vi "Check Main Measurement for Instrument Drivers.vi"(0 "Instrument containing subVIs":path[](array[path]), 5 "Measurement path":path, 11 "error in (no error)":errorcluster) -> (4 "Instrument containing subVIs Out":path[](array[path]), 15 "error out":errorcluster)   [LabVIEW 2021, in "Multiple Converter.lvlib"]
uses:
  Multiple Converter.lvlib
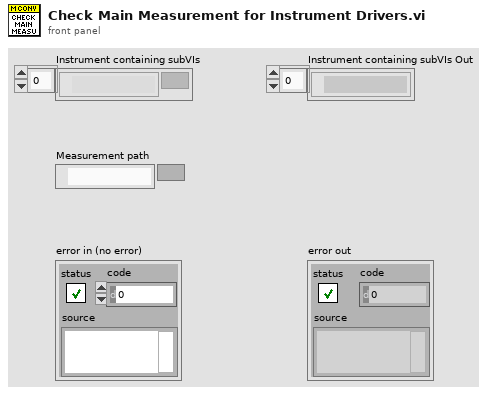
[diagram p1: front panel]
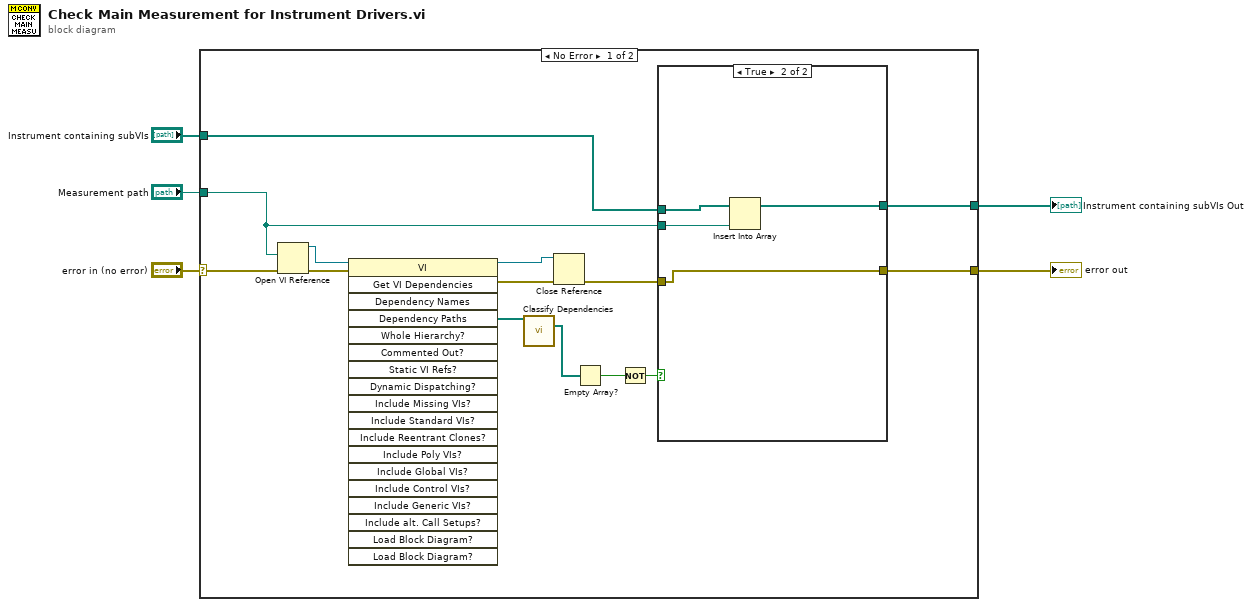
[diagram p0: block diagram]
diagram:
  n1 = case shown="No Error" "error in (no error)" {
    selector: "error in (no error)" -> [w16 w26]
    tunnel: [w6 w26] -> w5
    tunnel: "Measurement path" -> [w8 _]
    tunnel: "Instrument containing subVIs" -> [w9 _]
    tunnel: [w7 _] -> w1
    frame No Error {
      n2 = Open VI Reference(vi path=w8, error in (no error)=w16) -> (vi reference=w13:refnum<vi>, error out=w19:errorcluster)  [unwired: 4 in]
      n3 = invoke class="VI" method="Get VI Dependencies"(reference=w13, error in=w19) -> (reference out=w12:refnum<vi>, error out=w18:errorcluster, "Dependency Paths"=w17:path[])  [unwired: 17 in, 16 out]
      n4 = call "Classify Dependencies.vi"("Dependency paths"=w17) -> ("DriverVIs"=w14:path[])  [unwired: 13 in, 1 out]
      n5 = Close Reference(reference=w12, error in (no error)=w18) -> (error out=w11:errorcluster)
      n6 = Empty Array?(array=w14) -> (empty?=w15:bool)
      n7 = Not(x=w15) -> (.not. x?=w10:bool)
      n8 = case shown="True" w10 {
        tunnel: w11 -> [w21 w22]
        tunnel: w9 -> [w20 w25]
        tunnel: w8 -> [_ w24]
        tunnel: [w20 w23] -> w7
        tunnel: [w21 w22] -> w6
        frame False {
        }
        frame True {
          n9 = Insert Into Array(array=w25, new element=w24) -> (w23:path[])  [unwired: 1 in]
        }
      }
    }
    frame Error {
    }
  }
  "error out" <- w5
  "Instrument containing subVIs Out" <- w1
